vi "Periodic Tasks.vi"(8 "error in":errorcluster) -> ()   [LabVIEW 2019]
doc: "This VI runs in parallel to other tasks. It can contain as many user-defined periodic loops as you need. These can carry out PID or other sorts of timed response."
uses:
  <vilib>/Rock Robotics/WPI/ThirdParty/JAS_Junk/TrajLib/SWERVE_DRIVE_MODULE_STATE.ctl
  <vilib>/Rock Robotics/WPI/ThirdParty/JAS_Junk/TrajLib/ROTATION2D.ctl
  Robot Global Data.vi
  <vilib>/Rock Robotics/Network Tables/NT Write Number.vi
  <vilib>/Rock Robotics/Network Tables/NT Write Boolean.vi
  <vilib>/Rock Robotics/Network Tables/NT Write Numeric Array.vi
  <vilib>/Rock Robotics/Network Tables/NT Write Boolean Array.vi
  Secret_Control_Library_Protected/Secret_Control_Library_Protected.lvlib
  <vilib>/Rock Robotics/WPI/ThirdParty/JAS_Junk/TrajLib/Trajectory_Library.lvlib
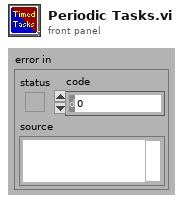
[diagram p1: front panel]
types:
  T1 = typedef "Trajectory_Library.lvlib/SWERVE_DRIVE_MODULE_STATE.ctl" = cluster{"Speed":dbl, "Angle":T2}
  T2 = typedef "Trajectory_Library.lvlib/ROTATION2D.ctl" = cluster{"VALUE":dbl, "COS":dbl, "SIN":dbl}
  T3 = typedef "SWERVE_MODULE_TYPDEF.ctl" = cluster{"SwervDriveMotor":T4, "SwerveSwerveMotor":T4, "SwerveDriveEnc":T9, "SwerveSwerveEnc":T9}
  T4 = typedef "WPI_MotorControlDeviceRef.ctl" = cluster{"DeviceStatus":errorcluster, "Type":T5, "PWM":cluster{"PWM Channel":T6, "DeadBand":T7}, "CAN":cluster{"Device Number":u8, "SetOutput VI Ref":variant, "GetOutput VI Ref":variant, "Enable VI Ref":variant, "Disable VI Ref":variant, "Data":variant}, "Invert":bool, "DIO PWM":cluster{"PWM \"Enable\" Channel":T6, "DIOChannel":T8, "PWM Rate":dbl}}
  T5 = typedef "WPI_MotorControlType.ctl" = enum16{"PWM", "CAN", "DIO PWM"}
  T6 = typedef "FPGA_DIOPWMChannel.ctl" = enum8{"PWM 0", "PWM 1", "PWM 2", "PWM 3", "PWM 4", "PWM 5", "PWM 6", "PWM 7", "PWM 8", "PWM 9", "PWM MXP 0", "PWM MXP 1", "PWM MXP 2", "PWM MXP 3", "PWM MXP 4", "PWM MXP 5", "PWM MXP 6", "PWM MXP 7", "PWM MXP 8", "PWM MXP 9", "Invalid"}
  T7 = typedef "WPI_PWMDeadband.ctl" = cluster{"Name":string, "maxPositivePwm":i32, "minPositivePwm":i32, "centerPwm":i32, "maxNegativePwm":i32, "minNegativePwm":i32, "angularRange":u16}
  T8 = typedef "FPGA_DIOChannel.ctl" = enum8{"DIO 0", "DIO 1", "DIO 2", "DIO 3", "DIO 4", "DIO 5", "DIO 6", "DIO 7", "DIO 8", "DIO 9", "DIO MXP 0", "DIO MXP 1", "DIO MXP 2", "DIO MXP 3", "DIO MXP 4", "DIO MXP 5", "DIO MXP 6", "DIO MXP 7", "DIO MXP 8", "DIO MXP 9", "DIO MXP 10", "DIO MXP 11", "DIO MXP 12", "DIO MXP 13", "DIO MXP 14", "DIO MXP 15", "SPI Port CS1", "SPI Port CS2", "SPI Port CS3", "SPI Port MISO", "SPI Port MOSI", "Invalid"}
  T9 = typedef "WPI_EncoderDevRef.ctl" = cluster{"DevStatus":errorcluster, "EncoderIndex":T10, "CounterIndex":T11, "DistancePerCount":dbl, "Decoding Type":T12}
  T10 = typedef "FPGA_EncoderIdx.ctl" = enum8{"Enc 0", "Enc 1", "Enc 2", "Enc 3", "Enc 4", "Enc 5", "Enc 6", "Enc 7", "Invalid"}
  T11 = typedef "FPGA_CounterCtrSystemIndex.ctl" = enum8{"Ctr 0", "Ctr 1", "Ctr 2", "Ctr 3", "Ctr 4", "Ctr 5", "Ctr 6", "Ctr 7", "Invalid"}
  T12 = typedef "WPI_EncoderType.ctl" = enum16{"1x", "2x", "4x"}
  T13 = typedef "Trajectory_Library.lvlib/SWERVE_DRIVE_KINEMATICS.ctl" = cluster{"NumModules":i32, "InverseKinematics":T14, "ForwardKinematics":T14, "Modules":T15[], "PrevCoR":T15}
  T14 = typedef "NI_Matrix.lvlib/RealMatrix.ctl" = dbl[][]
  T15 = typedef "Trajectory_Library.lvlib/TRANSLATION2D.ctl" = cluster{"X":dbl, "Y":dbl}
  T16 = typedef "WPI_GyroDevRef.ctl" = cluster{"DevStatus":errorcluster, "Analog Channel":T17, "Gain (VoltsPerDegree/Second)":dbl, "Gyro Type":enum16{"Analog", "XRS450"}, "Handle":i32, "SPI Bus":T18, "Device Found":bool, "Sample Rate":dbl, "Calibrate On Open":bool, "Offset":dbl}
  T17 = typedef "FPGA_AIChannel.ctl" = enum8{"AI 0", "AI 1", "AI 2", "AI 3", "AI MXP 0", "AI MXP 1", "AI MXP 2", "AI MXP 3", "Invalid"}
  T18 = typedef "spi_bus.ctl" = enum16{"SPI On-Board, CS0", "SPI On-Board, CS1", "SPI On-Board, CS2", "SPI On-Board, CS3", "SPI MXP", "Invalid"}
  T19 = typedef "Trajectory_Library.lvlib/SWERVE_DRIVE_ODOMETRY.ctl" = cluster{"POSE":T20, "GyroOffset":T2, "PreviousAngle":T2, "PrevTime":dbl}
  T20 = typedef "Trajectory_Library.lvlib/POSE2D.ctl" = cluster{"TRANSLATION":T15, "ROTATION":T2}
  T21 = typedef "Trajectory_Library.lvlib/CHASSIS_SPEEDS.ctl" = cluster{"vX":dbl, "vY":dbl, "vOmega":dbl}
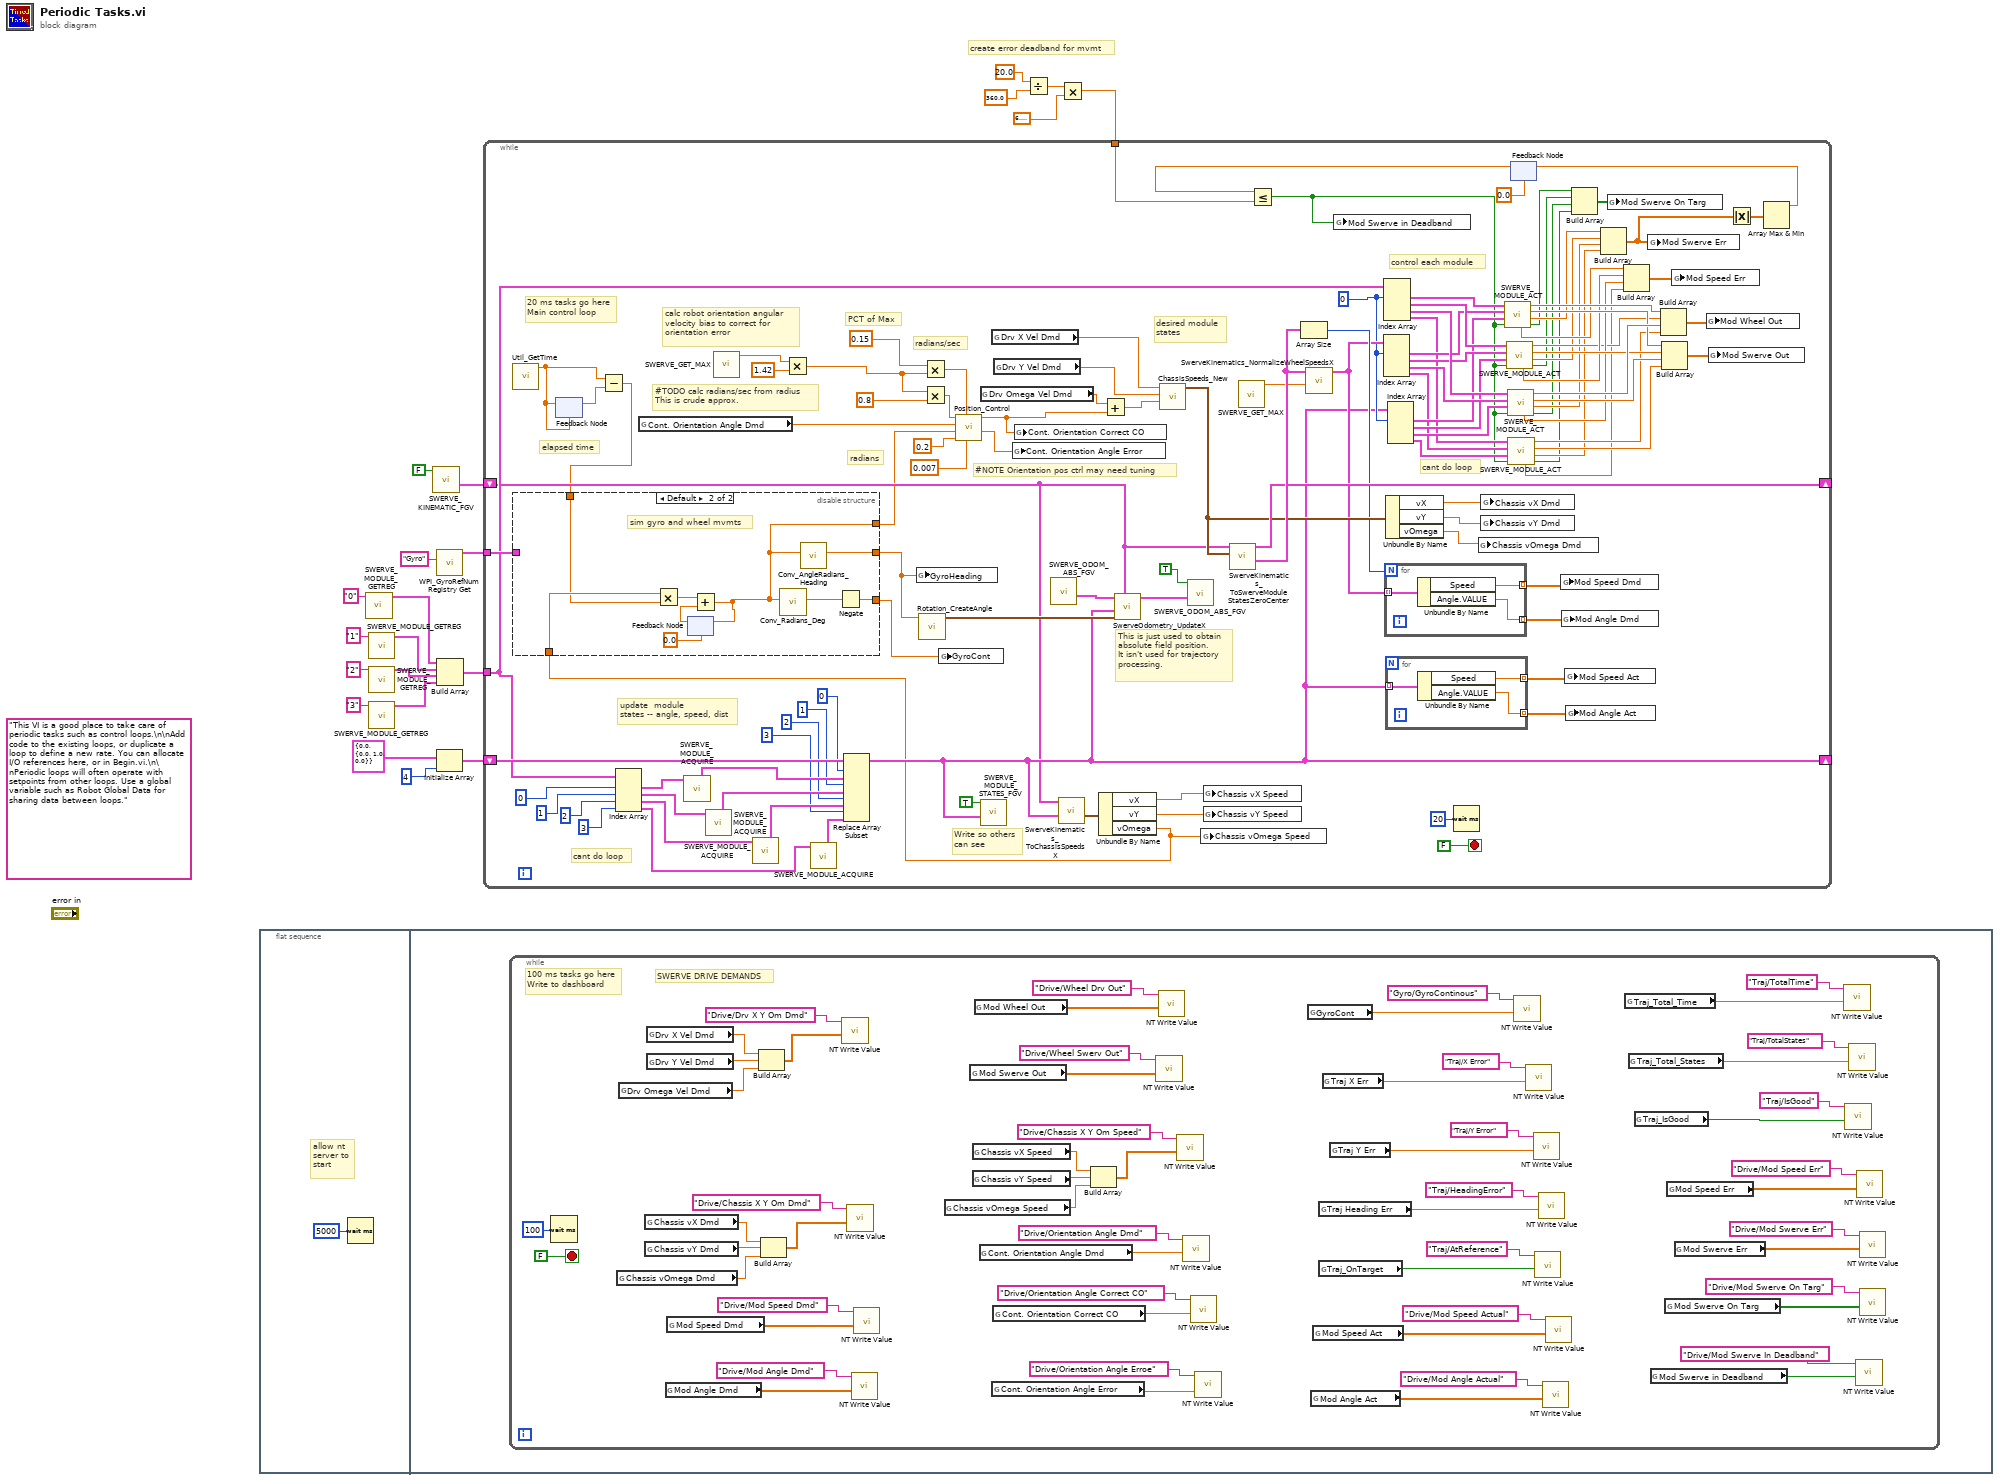
[diagram p0: block diagram]
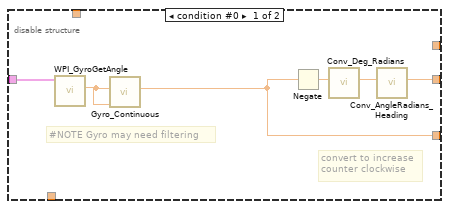
[diagram p2: hidden frame]
diagram:
  (unwired) "This VI is a good place to take care of periodic tasks such as control loops.\n\nAdd code to the existing loops, or duplicate a loop to define a new rate. You can allocate I/O references here, or in Begin.vi.\n\nPeriodic loops will often operate with setpoints from other loops. Use a global variable such as Robot Global Data for sharing data between loops."
  # "create error deadband for mvmt"
  n1 = flat-sequence {
    frame #0 {
      # "allow nt\nserver to \nstart"
      n2 = Wait (ms)(milliseconds to wait=u32 5000) -> ()  [unwired: 1 out]
    }
    frame #1 {
      n3 = while {
        stop <- FALSE stop-if-true
        # "SWERVE DRIVE DEMANDS"
        # "100 ms tasks go here\nWrite to dashboard"
        n4 = Wait (ms)(milliseconds to wait=u32 100) -> ()  [unwired: 1 out]
        n5 = global read "Robot Global Data.vi" "Chassis vOmega Dmd"() -> (w55:dbl)
        n6 = global read "Robot Global Data.vi" "Drv Omega Vel Dmd"() -> (w60:dbl)
        n7 = global read "Robot Global Data.vi" "Chassis vX Dmd"() -> (w53:dbl)
        n8 = global read "Robot Global Data.vi" "Chassis vY Dmd"() -> (w54:dbl)
        n9 = global read "Robot Global Data.vi" "Drv X Vel Dmd"() -> (w58:dbl)
        n10 = global read "Robot Global Data.vi" "Drv Y Vel Dmd"() -> (w59:dbl)
        n11 = global read "Robot Global Data.vi" "Mod Angle Dmd"() -> (w48:dbl[])
        n12 = global read "Robot Global Data.vi" "Mod Speed Dmd"() -> (w50:dbl[])
        n13 = Build Array(w58, w59, w60) -> (w57:dbl[])
        n14 = Build Array(w53, w54, w55) -> (w52:dbl[])
        n15 = call-poly <vilib>:"NT Write Value.vi"("Numeric Array"=w57, "Name"="Drive/Drv X Y Om Dmd") -> ()  [unwired: 9 in, 1 out]
        n16 = call-poly <vilib>:"NT Write Value.vi"("Numeric Array"=w52, "Name"="Drive/Chassis X Y Om Dmd") -> ()  [unwired: 9 in, 1 out]
        n17 = call-poly <vilib>:"NT Write Value.vi"("Numeric Array"=w48, "Name"="Drive/Mod Angle Dmd") -> ()  [unwired: 9 in, 1 out]
        n18 = call-poly <vilib>:"NT Write Value.vi"("Numeric Array"=w50, "Name"="Drive/Mod Speed Dmd") -> ()  [unwired: 9 in, 1 out]
        n19 = global read "Robot Global Data.vi" "Chassis vOmega Speed"() -> (w38:dbl)
        n20 = global read "Robot Global Data.vi" "Mod Swerve Out"() -> (w40:dbl[])
        n21 = global read "Robot Global Data.vi" "Chassis vX Speed"() -> (w36:dbl)
        n22 = global read "Robot Global Data.vi" "Chassis vY Speed"() -> (w37:dbl)
        n23 = global read "Robot Global Data.vi" "Mod Wheel Out"() -> (w42:dbl[])
        n24 = global read "Robot Global Data.vi" "Cont. Orientation Angle Dmd"() -> (w61:dbl)
        n25 = global read "Robot Global Data.vi" "Cont. Orientation Angle Error"() -> (w32:dbl)
        n26 = global read "Robot Global Data.vi" "Cont. Orientation Correct CO"() -> (w31:dbl)
        n27 = Build Array(w36, w37, w38) -> (w35:dbl[])
        n28 = call-poly <vilib>:"NT Write Value.vi"("Numeric Array"=w40, "Name"="Drive/Wheel Swerv Out") -> ()  [unwired: 9 in, 1 out]
        n29 = call-poly <vilib>:"NT Write Value.vi"("Numeric Array"=w42, "Name"="Drive/Wheel Drv Out") -> ()  [unwired: 9 in, 1 out]
        n30 = call-poly <vilib>:"NT Write Value.vi"("Numeric Array"=w35, "Name"="Drive/Chassis X Y Om Speed") -> ()  [unwired: 9 in, 1 out]
        n31 = call-poly <vilib>:"NT Write Value.vi"("Numeric"=w61, "Name"="Drive/Orientation Angle Dmd") -> ()  [unwired: 9 in, 1 out]
        n32 = call-poly <vilib>:"NT Write Value.vi"("Numeric"=w31, "Name"="Drive/Orientation Angle Correct CO") -> ()  [unwired: 9 in, 1 out]
        n33 = call-poly <vilib>:"NT Write Value.vi"("Numeric"=w32, "Name"="Drive/Orientation Angle Erroe") -> ()  [unwired: 9 in, 1 out]
        n34 = global read "Robot Global Data.vi" "GyroCont"() -> (w78:dbl)
        n35 = global read "Robot Global Data.vi" "Mod Angle Act"() -> (w44:dbl[])
        n36 = global read "Robot Global Data.vi" "Mod Speed Act"() -> (w46:dbl[])
        n37 = global read "Robot Global Data.vi" "Traj Heading Err"() -> (w72:dbl)
        n38 = global read "Robot Global Data.vi" "Traj_OnTarget"() -> (w70:bool)
        n39 = global read "Robot Global Data.vi" "Traj X Err"() -> (w76:dbl)
        n40 = global read "Robot Global Data.vi" "Traj Y Err"() -> (w74:dbl)
        n41 = call-poly <vilib>:"NT Write Value.vi"("Numeric"=w78, "Name"="Gyro/GyroContinous") -> ()  [unwired: 9 in, 1 out]
        n42 = call-poly <vilib>:"NT Write Value.vi"("Numeric"=w76, "Name"="Traj/X Error") -> ()  [unwired: 9 in, 1 out]
        n43 = call-poly <vilib>:"NT Write Value.vi"("Numeric"=w74, "Name"="Traj/Y Error") -> ()  [unwired: 9 in, 1 out]
        n44 = call-poly <vilib>:"NT Write Value.vi"("Boolean"=w70, "Name"="Traj/AtReference") -> ()  [unwired: 9 in, 1 out]
        n45 = call-poly <vilib>:"NT Write Value.vi"("Numeric"=w72, "Name"="Traj/HeadingError") -> ()  [unwired: 9 in, 1 out]
        n46 = call-poly <vilib>:"NT Write Value.vi"("Numeric Array"=w44, "Name"="Drive/Mod Angle Actual") -> ()  [unwired: 9 in, 1 out]
        n47 = call-poly <vilib>:"NT Write Value.vi"("Numeric Array"=w46, "Name"="Drive/Mod Speed Actual") -> ()  [unwired: 9 in, 1 out]
        n48 = global read "Robot Global Data.vi" "Traj_Total_Time"() -> (w68:dbl)
        n49 = global read "Robot Global Data.vi" "Traj_Total_States"() -> (w66:dbl)
        n50 = global read "Robot Global Data.vi" "Traj_IsGood"() -> (w64:bool)
        n51 = global read "Robot Global Data.vi" "Mod Swerve in Deadband"() -> (w24:bool)
        n52 = global read "Robot Global Data.vi" "Mod Swerve On Targ"() -> (w25:bool[])
        n53 = global read "Robot Global Data.vi" "Mod Speed Err"() -> (w27:dbl[])
        n54 = global read "Robot Global Data.vi" "Mod Swerve Err"() -> (w26:dbl[])
        n55 = call-poly <vilib>:"NT Write Value.vi"("Numeric"=w68, "Name"="Traj/TotalTime") -> ()  [unwired: 9 in, 1 out]
        n56 = call-poly <vilib>:"NT Write Value.vi"("Boolean"=w64, "Name"="Traj/IsGood") -> ()  [unwired: 9 in, 1 out]
        n57 = call-poly <vilib>:"NT Write Value.vi"("Numeric"=w66, "Name"="Traj/TotalStates") -> ()  [unwired: 9 in, 1 out]
        n58 = call-poly <vilib>:"NT Write Value.vi"("Boolean"=w24, "Name"="Drive/Mod Swerve In Deadband") -> ()  [unwired: 9 in, 1 out]
        n59 = call-poly <vilib>:"NT Write Value.vi"("Numeric Array"=w27, "Name"="Drive/Mod Speed Err") -> ()  [unwired: 9 in, 1 out]
        n60 = call-poly <vilib>:"NT Write Value.vi"("Numeric Array"=w26, "Name"="Drive/Mod Swerve Err") -> ()  [unwired: 9 in, 1 out]
        n61 = call-poly <vilib>:"NT Write Value.vi"("Boolean Array"=w25, "Name"="Drive/Mod Swerve On Targ") -> ()  [unwired: 9 in, 1 out]
      }
    }
  }
  n62 = call "SWERVE_MODULE_GETREG.vi"("Suffix"="0" ("NameSuffix")) -> ("Swerve Module TypDef"=w14:T3)  [unwired: 10 in]
  n63 = call "SWERVE_MODULE_GETREG.vi"("Suffix"="1" ("NameSuffix")) -> ("Swerve Module TypDef"=w13:T3)  [unwired: 10 in]
  n64 = call "SWERVE_MODULE_GETREG.vi"("Suffix"="2" ("NameSuffix")) -> ("Swerve Module TypDef"=w12:T3)  [unwired: 10 in]
  n65 = call "SWERVE_MODULE_GETREG.vi"("Suffix"="3" ("NameSuffix")) -> ("Swerve Module TypDef"=w6:T3)  [unwired: 10 in]
  n66 = call "SWERVE_KINEMATIC_FGV.vi"("WRITE"=FALSE) -> ("out SWERVE_DRIVE_KINEMATICS"=w18:T13)  [unwired: 10 in]
  n67 = call <vilib>:"WPI_GyroRefNum Registry Get.vi"("refnum name"="Gyro") -> ("GyroDevRef"=w8:T16)  [unwired: 9 in, 1 out]
  n68 = Initialize Array(T1 {"Speed"=0.0, "Angle"={"VALUE"=0.0, "COS"=1.0, "SIN"=0.0}} ("SWERVE_DRIVE_MODULE_STATE"), 4 ("dimension size")) -> (w19:T1[])
  n69 = Build Array(w14, w13, w12, w6) -> (w11:T3[])
  n70 = Divide(x=20.0, y=360.0) -> (x/y=w3:dbl)
  n71 = Multiply(x=w3, y=6.283185307179586) -> (x*y=w1:dbl)
  n72 = while {
    shift-right: [w132] -> _
    shift-left: w19 -> [w163]
    tunnel: w11 -> [w157]
    shift-right: [w178] -> _
    shift-left: w18 -> [w131]
    tunnel: w8 -> [w175]
    tunnel: w1 -> [w83]
    stop <- FALSE stop-if-true
    w135 = 0 ("index")
    # "#TODO calc radians/sec from radius\nThis is crude approx."
    # "PCT of Max"
    # "This is just used to obtain\nabsolute field position.\nIt isn't used for trajectory\nprocessing."
    # "Write so others\ncan see"
    # "#NOTE Orientation pos ctrl may need tuning"
    # "elapsed time"
    # "cant do loop"
    # "cant do loop"
    # "control each module"
    # "update  module\nstates -- angle, speed, dist"
    # "desired module\nstates"
    # "radians/sec"
    # "radians"
    # "calc robot orientation angular\nvelocity bias to correct for\norientation error"
    # "20 ms tasks go here\nMain control loop"
    n73 = call <vilib>:"Util_GetTime.vi"() -> ("FPGA_Time_Seconds"=w118:dbl)  [unwired: 10 in, 1 out]
    n74 = feedback #1(w118) -> (w119:dbl)
    n75 = feedback-in #1(w118) -> ()
    n76 = Subtract(x=w118, y=w119) -> (x-y=w117:dbl)
    n77 = Index Array(array=w157, index #1=0 ("index"), index #2=1 ("index"), index #3=2 ("index"), index #4=3 ("index")) -> (element #1=w160:T3, element #2=w159:T3, element #3=w158:T3, element #4=w122:T3)
    n78 = global read "Robot Global Data.vi" "Cont. Orientation Angle Dmd"() -> (w89:dbl)
    n79 = call "SWERVE_MODULE_ACQUIRE.vi"("Swerve Module TypDef"=w160) -> ("Swerve Module State"=w164:T1)  [unwired: 5 in, 5 out]
    n80 = call "SWERVE_MODULE_ACQUIRE.vi"("Swerve Module TypDef"=w159) -> ("Swerve Module State"=w161:T1)  [unwired: 5 in, 5 out]
    n81 = call "SWERVE_GET_MAX.vi"() -> ("Max Wheel Vel (Meter/Sec)"=w94:dbl)  [unwired: 10 in, 1 out]
    n82 = call "SWERVE_MODULE_ACQUIRE.vi"("Swerve Module TypDef"=w158) -> ("Swerve Module State"=w162:T1)  [unwired: 5 in, 5 out]
    n83 = Multiply(x=w94, y=1.42) -> (x*y=w92:dbl)
    n84 = call "SWERVE_MODULE_ACQUIRE.vi"("Swerve Module TypDef"=w122) -> ("Swerve Module State"=w121:T1)  [unwired: 5 in, 5 out]
    n85 = Replace Array Subset(array=w163, new element #1=w164, index #1=0 ("index"), new element #2=w161, index #2=1 ("index"), new element #3=w162, index #3=2 ("index"), new element #4=w121, index #4=3 ("index")) -> (w132:T1[])
    n86 = Multiply(x=0.15, y=w92) -> (x*y=w186:dbl)
    n87 = Multiply(x=w92, y=0.8) -> (x*y=w116:dbl)
    n88 = global read "Robot Global Data.vi" "Drv Omega Vel Dmd"() -> (w182:dbl)
    n89 = call "SWERVE_MODULE_STATES_FGV.vi"("in Current Module States"=w132, "WRITE"=TRUE) -> ()  [unwired: 9 in, 1 out]
    n90 = global read "Robot Global Data.vi" "Drv X Vel Dmd"() -> (w181:dbl)
    n91 = global read "Robot Global Data.vi" "Drv Y Vel Dmd"() -> (w180:dbl)
    n92 = call "SWERVE_ODOM_ABS_FGV.vi"() -> ("out SWERVE_DRIVE_ODOMETRY"=w190:T19)  [unwired: 11 in]
    n93 = call <vilib>:"SwerveKinematics_ToChassisSpeedsX.vi"("WheelStates"=w132, "in SWERVE_DRIVE_KINEMATICS"=w131) -> ("Chassis Speed"=w133:T21)  [unwired: 9 in]
    n94 = Unbundle By Name(w133) -> ("vX"=w130:dbl, "vY"=w129:dbl, "vOmega"=w128:dbl)
    n95 = disable-structure shown="Default" {
      disable-tunnel: [w202 w210] -> w91
      disable-tunnel: [w200 w209] -> w176
      disable-tunnel: w175 -> [w199 _]
      disable-tunnel: w128 -> [_ w208]
      disable-tunnel: w117 -> [_ w206]
      disable-tunnel: [_ w205] -> w90
      frame condition #0 {
        # "#NOTE Gyro may need filtering"
        # "convert to increase\ncounter clockwise"
        n96 = call <vilib>:"WPI_GyroGetAngle.vi"("GyroDevRef"=w199) -> ("Angle"=w201:dbl)  [unwired: 7 in, 3 out]
        n97 = call "Gyro_Continuous.vi"("GyroInitial"=w201, "GyroInput"=w201) -> ("GyroContinuous"=w200:dbl)  [unwired: 9 in]
        n98 = Negate(x=w200) -> (-x=w203:dbl)
        n99 = call <vilib>:"Conv_Deg_Radians.vi"("Degress"=w203) -> ("Radians"=w204:dbl)  [unwired: 10 in]
        n100 = call <vilib>:"Conv_AngleRadians_Heading.vi"("Radians"=w204) -> ("Heading"=w202:dbl)  [unwired: 10 in]
      }
      frame condition #1 (active) {
        # "sim gyro and wheel mvmts"
        n101 = Multiply(x=w208, y=w206) -> (x*y=w211:dbl)
        n102 = feedback #2(0.0) -> (w212:dbl)
        n103 = Add(x=w211, y=w212) -> (x+y=w205:dbl)
        n104 = feedback-in #2(w205) -> ()
        n105 = call <vilib>:"Conv_Radians_Deg.vi"("Radians"=w205) -> ("Degrees"=w207:dbl)  [unwired: 10 in]
        n106 = call <vilib>:"Conv_AngleRadians_Heading.vi"("Radians"=w205) -> ("Heading"=w210:dbl)  [unwired: 10 in]
        n107 = Negate(x=w207) -> (-x=w209:dbl)
      }
    }
    n108 = global write "Robot Global Data.vi" "GyroHeading"(w91) -> ()
    n109 = call <vilib>:"Rotation_CreateAngle.vi"("Angle"=w91) -> ("ROTATION"=w189:T2)  [unwired: 10 in]
    n110 = global write "Robot Global Data.vi" "GyroCont"(w176) -> ()
    n111 = call "Position_Control.vi"("ErrDeadband"=0.007, "MinOutput"=w186, "ErrThreshold"=0.2, "CurrentPosition"=w90, "TargetPosition"=w89, "MaxOutput"=w116) -> ("PositionError"=w110:dbl, "Output"=w111:dbl)  [unwired: 3 in, 1 out]
    n112 = global write "Robot Global Data.vi" "Cont. Orientation Angle Error"(w110) -> ()
    n113 = global write "Robot Global Data.vi" "Cont. Orientation Correct CO"(w111) -> ()
    n114 = Add(x=w182, y=w111) -> (x+y=w134:dbl)
    n115 = call <vilib>:"SwerveOdometry_UpdateX.vi"("SWERVE_DRIVE_KINEMATICS"=w131, "gyroAngle"=w189, "module States"=w132, "in SWERVE_DRIVE_ODOMETRY"=w190) -> ("out SWERVE_DRIVE_ODOMETRY"=w187:T19)  [unwired: 6 in, 1 out]
    n116 = call <vilib>:"ChassisSpeeds_New.vi"("vAngular"=w134, "vY"=w180, "vX"=w181) -> ("CHASSIS"=w173:T21)  [unwired: 8 in]
    n117 = call "SWERVE_ODOM_ABS_FGV.vi"("in SWERVE_DRIVE_ODOMETRY"=w187, "WRITE"=TRUE) -> ()  [unwired: 9 in, 1 out]
    n118 = global write "Robot Global Data.vi" "Chassis vOmega Speed"(w128) -> ()
    n119 = global write "Robot Global Data.vi" "Chassis vX Speed"(w130) -> ()
    n120 = global write "Robot Global Data.vi" "Chassis vY Speed"(w129) -> ()
    n121 = call <vilib>:"SwerveKinematics_ToSwerveModuleStatesZeroCenter.vi"("ChassisSpeeds"=w173, "in SWERVE_DRIVE_KINEMATICS"=w131) -> ("ModuleStates"=w179:T1[], "out SWERVE_DRIVE_KINEMATICS"=w178:T13)  [unwired: 8 in]
    n122 = call "SWERVE_GET_MAX.vi"() -> ("Max Wheel Vel (Meter/Sec)"=w174:dbl)  [unwired: 10 in, 1 out]
    n123 = Array Size(array=w179) -> (size(s)=w169:i32)
    n124 = call <vilib>:"SwerveKinematics_NormalizeWheelSpeedsX.vi"("AttainableMaxSpeed"=w174, "in WheelStates"=w179) -> ("out WheelStates"=w153:T1[])  [unwired: 9 in]
    n125 = Index Array(array=w153, index #1=w135) -> (element #1=w152:T1, element #2=w151:T1, element #3=w150:T1, element #4=w124:T1)  [unwired: 3 in]
    n126 = Index Array(array=w157, index #1=w135) -> (element #1=w156:T3, element #2=w155:T3, element #3=w154:T3, element #4=w125:T3)  [unwired: 3 in]
    n127 = for {
      N: w169 -> [_]
      tunnel: w153 -> [w198] mode=indexing
      tunnel: [w197] -> w168 mode=indexing
      tunnel: [w196] -> w167 mode=indexing
      n128 = Unbundle By Name(w198) -> ("Speed"=w196:dbl, "Angle.VALUE"=w197:dbl)
    }
    n129 = Unbundle By Name(w173) -> ("vX"=w172:dbl, "vY"=w171:dbl, "vOmega"=w170:dbl)
    n130 = for {
      tunnel: w132 -> [w195] mode=indexing
      tunnel: [w194] -> w165 mode=indexing
      tunnel: [w193] -> w166 mode=indexing
      n131 = Unbundle By Name(w195) -> ("Speed"=w193:dbl, "Angle.VALUE"=w194:dbl)
    }
    n132 = Index Array(array=w132, index #1=w135) -> (element #1=w149:T1, element #2=w148:T1, element #3=w147:T1, element #4=w123:T1)  [unwired: 3 in]
    n133 = Wait (ms)(milliseconds to wait=u32 20) -> ()  [unwired: 1 out]
    n134 = global write "Robot Global Data.vi" "Chassis vOmega Dmd"(w170) -> ()
    n135 = global write "Robot Global Data.vi" "Chassis vX Dmd"(w172) -> ()
    n136 = global write "Robot Global Data.vi" "Chassis vY Dmd"(w171) -> ()
    n137 = feedback #3(0.0) -> (w84:dbl)
    n138 = Less Or Equal?(x=w84, y=w83) -> (x <= y?=w82:bool)
    n139 = global write "Robot Global Data.vi" "Mod Swerve in Deadband"(w82) -> ()
    n140 = call "SWERVE_MODULE_ACT.vi"("SwervePosInDeadband"=w82, "Swerve Sense"=w149, "Swerve Dmd"=w152, "Swerve Module TypDef"=w156) -> ("SwerveOnTarget"=w98:bool, "SwervePosError"=w104:dbl, "Swerve Motor Dmd"=w143:dbl, "Wheel Motor Dmd"=w146:dbl, "WheelSpeedErr"=w108:dbl)  [unwired: 3 in]
    n141 = call "SWERVE_MODULE_ACT.vi"("SwervePosInDeadband"=w82, "Swerve Sense"=w148, "Swerve Dmd"=w151, "Swerve Module TypDef"=w155) -> ("SwerveOnTarget"=w97:bool, "SwervePosError"=w103:dbl, "Swerve Motor Dmd"=w142:dbl, "Wheel Motor Dmd"=w105:dbl, "WheelSpeedErr"=w107:dbl)  [unwired: 3 in]
    n142 = call "SWERVE_MODULE_ACT.vi"("SwervePosInDeadband"=w82, "Swerve Sense"=w147, "Swerve Dmd"=w150, "Swerve Module TypDef"=w154) -> ("SwerveOnTarget"=w96:bool, "SwervePosError"=w102:dbl, "Swerve Motor Dmd"=w141:dbl, "Wheel Motor Dmd"=w145:dbl, "WheelSpeedErr"=w106:dbl)  [unwired: 3 in]
    n143 = call "SWERVE_MODULE_ACT.vi"("SwervePosInDeadband"=w82, "Swerve Sense"=w123, "Swerve Dmd"=w124, "Swerve Module TypDef"=w125) -> ("SwerveOnTarget"=w95:bool, "SwervePosError"=w101:dbl, "Swerve Motor Dmd"=w126:dbl, "Wheel Motor Dmd"=w127:dbl, "WheelSpeedErr"=w100:dbl)  [unwired: 3 in]
    n144 = global write "Robot Global Data.vi" "Mod Speed Dmd"(w167) -> ()
    n145 = global write "Robot Global Data.vi" "Mod Angle Dmd"(w168) -> ()
    n146 = global write "Robot Global Data.vi" "Mod Speed Act"(w166) -> ()
    n147 = global write "Robot Global Data.vi" "Mod Angle Act"(w165) -> ()
    n148 = Build Array(w98, w97, w96, w95) -> (w99:bool[])
    n149 = Build Array(w104, w103, w102, w101) -> (w87:dbl[])
    n150 = global write "Robot Global Data.vi" "Mod Swerve On Targ"(w99) -> ()
    n151 = Build Array(w108, w107, w106, w100) -> (w109:dbl[])
    n152 = global write "Robot Global Data.vi" "Mod Swerve Err"(w87) -> ()
    n153 = Build Array(w146, w105, w145, w127) -> (w144:dbl[])
    n154 = Build Array(w143, w142, w141, w126) -> (w140:dbl[])
    n155 = global write "Robot Global Data.vi" "Mod Speed Err"(w109) -> ()
    n156 = global write "Robot Global Data.vi" "Mod Wheel Out"(w144) -> ()
    n157 = global write "Robot Global Data.vi" "Mod Swerve Out"(w140) -> ()
    n158 = Absolute Value(x=w87) -> (abs(x)=w88:dbl[])
    n159 = Array Max & Min(array=w88) -> (max value=w86:dbl)  [unwired: 3 out]
    n160 = feedback-in #3(w86) -> ()
  }
